vi "prototype_terminal.vi"() -> ()   [LabVIEW 2015]
uses:
  <vilib>/Analysis/baseanly.llb/Mean (DBL).vi
  <vilib>/Instr/_visa.llb/VISA Configure Serial Port (Instr).vi
  <vilib>/Analysis/NI_AALBase.lvlib
panel:
  in  "Tab Control":T1(tab)
  in  "Select channel":T2
  out "Current values":cluster{dbl, dbl, dbl, dbl}(graph)
  out "Error thermometer":bool
  out "Error pressure":bool
  out "Error amperage":bool
  out "Error voltage":bool
  out "SMA":cluster{dbl, dbl, dbl, dbl}(graph)
  in  "Clear":bool
  out "Amperage,A":dbl(slide) scale=0.0..2.5
  out "Pressure, kPa":dbl(knob) scale=0.0..50.0
  out "Thermometer, °C":dbl(slide) scale=0.0..60.0
  out "Voltage,V":dbl(knob) scale=0.0..5.0 scale format="%_2f"
  out "Voltage":dbl(graph)
  in  "Set voltage":sgl(knob) min=1 max=5 step=0.01 scale=0.0..5.0 scale format="%#.2f"
  out "Output voltage,V":dbl(knob) scale=1.0..5.0 scale format="%_2f"
  out "Received bytes":dbl
  in  "VISA resource name":refnum<visa-resource-name>
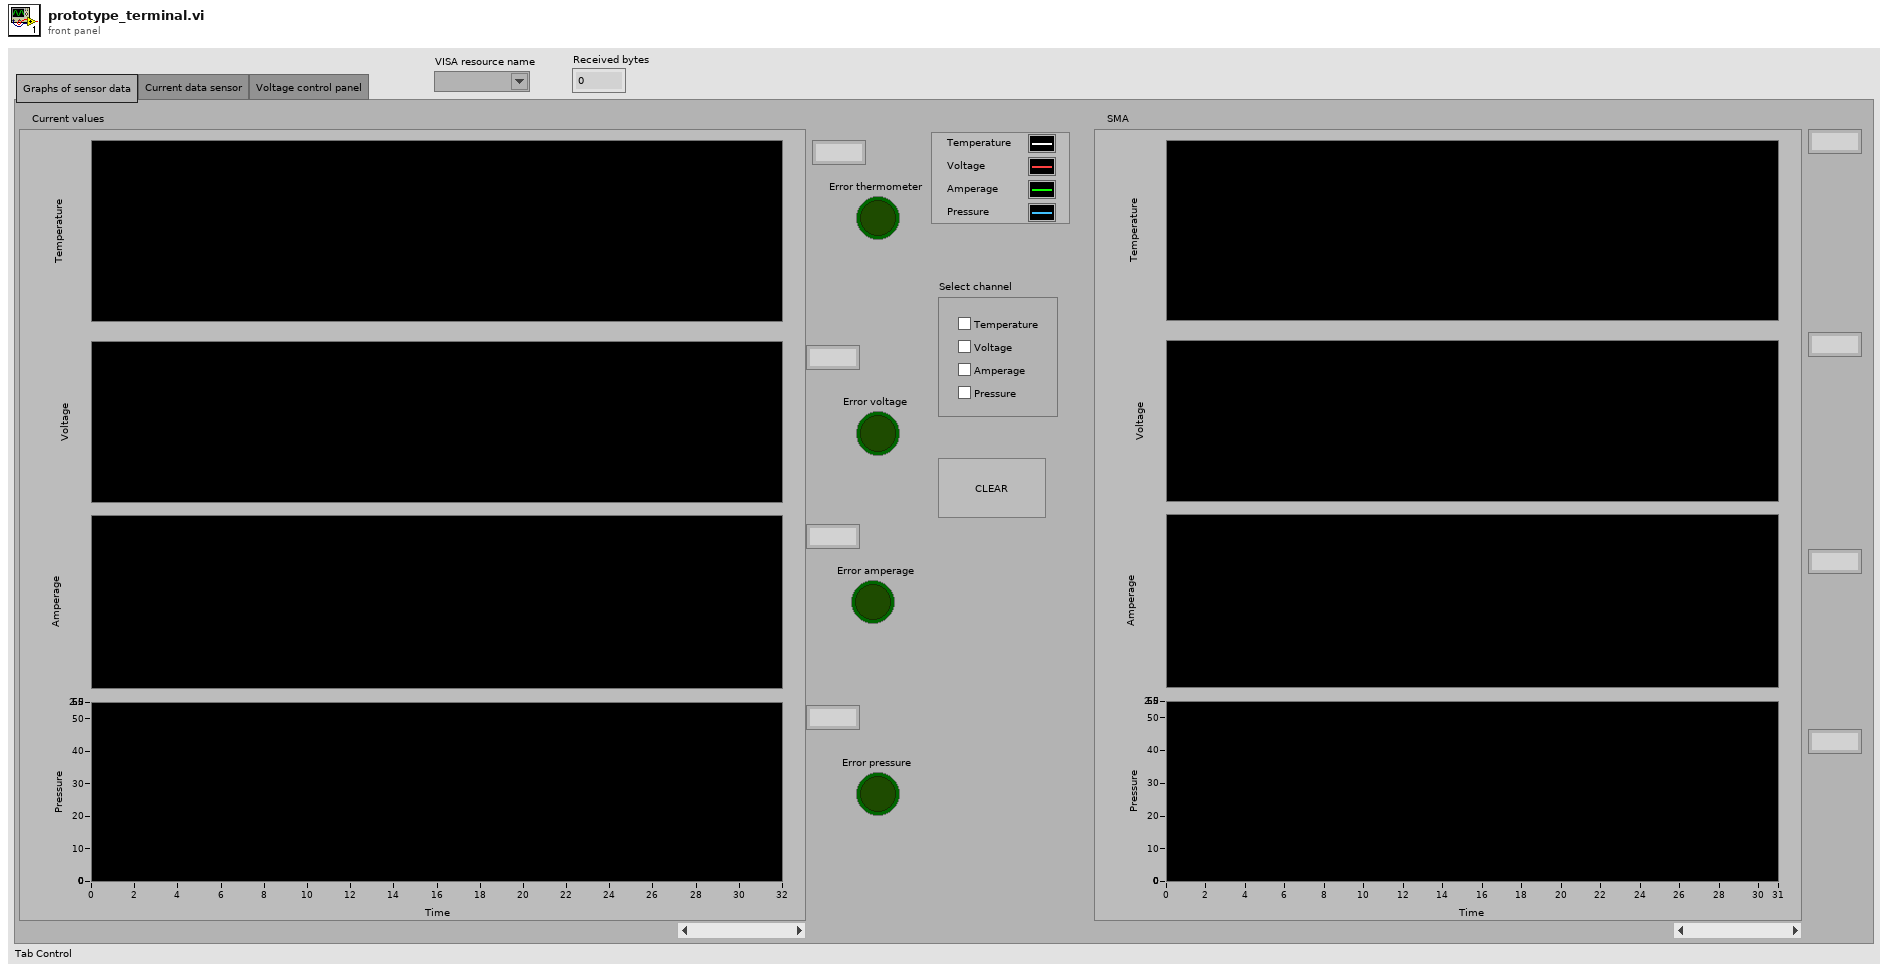
[diagram p1: front panel]
types:
  T1 = enum32{"Graphs of sensor data", "Current data sensor", "Voltage control panel"}
  T2 = cluster{"Ch1":bool, "Ch2":bool, "Ch3":bool, "Ch3 2":bool}
  T3 = cluster{"mean":dbl, "mean":dbl, "mean":dbl, "mean":dbl}
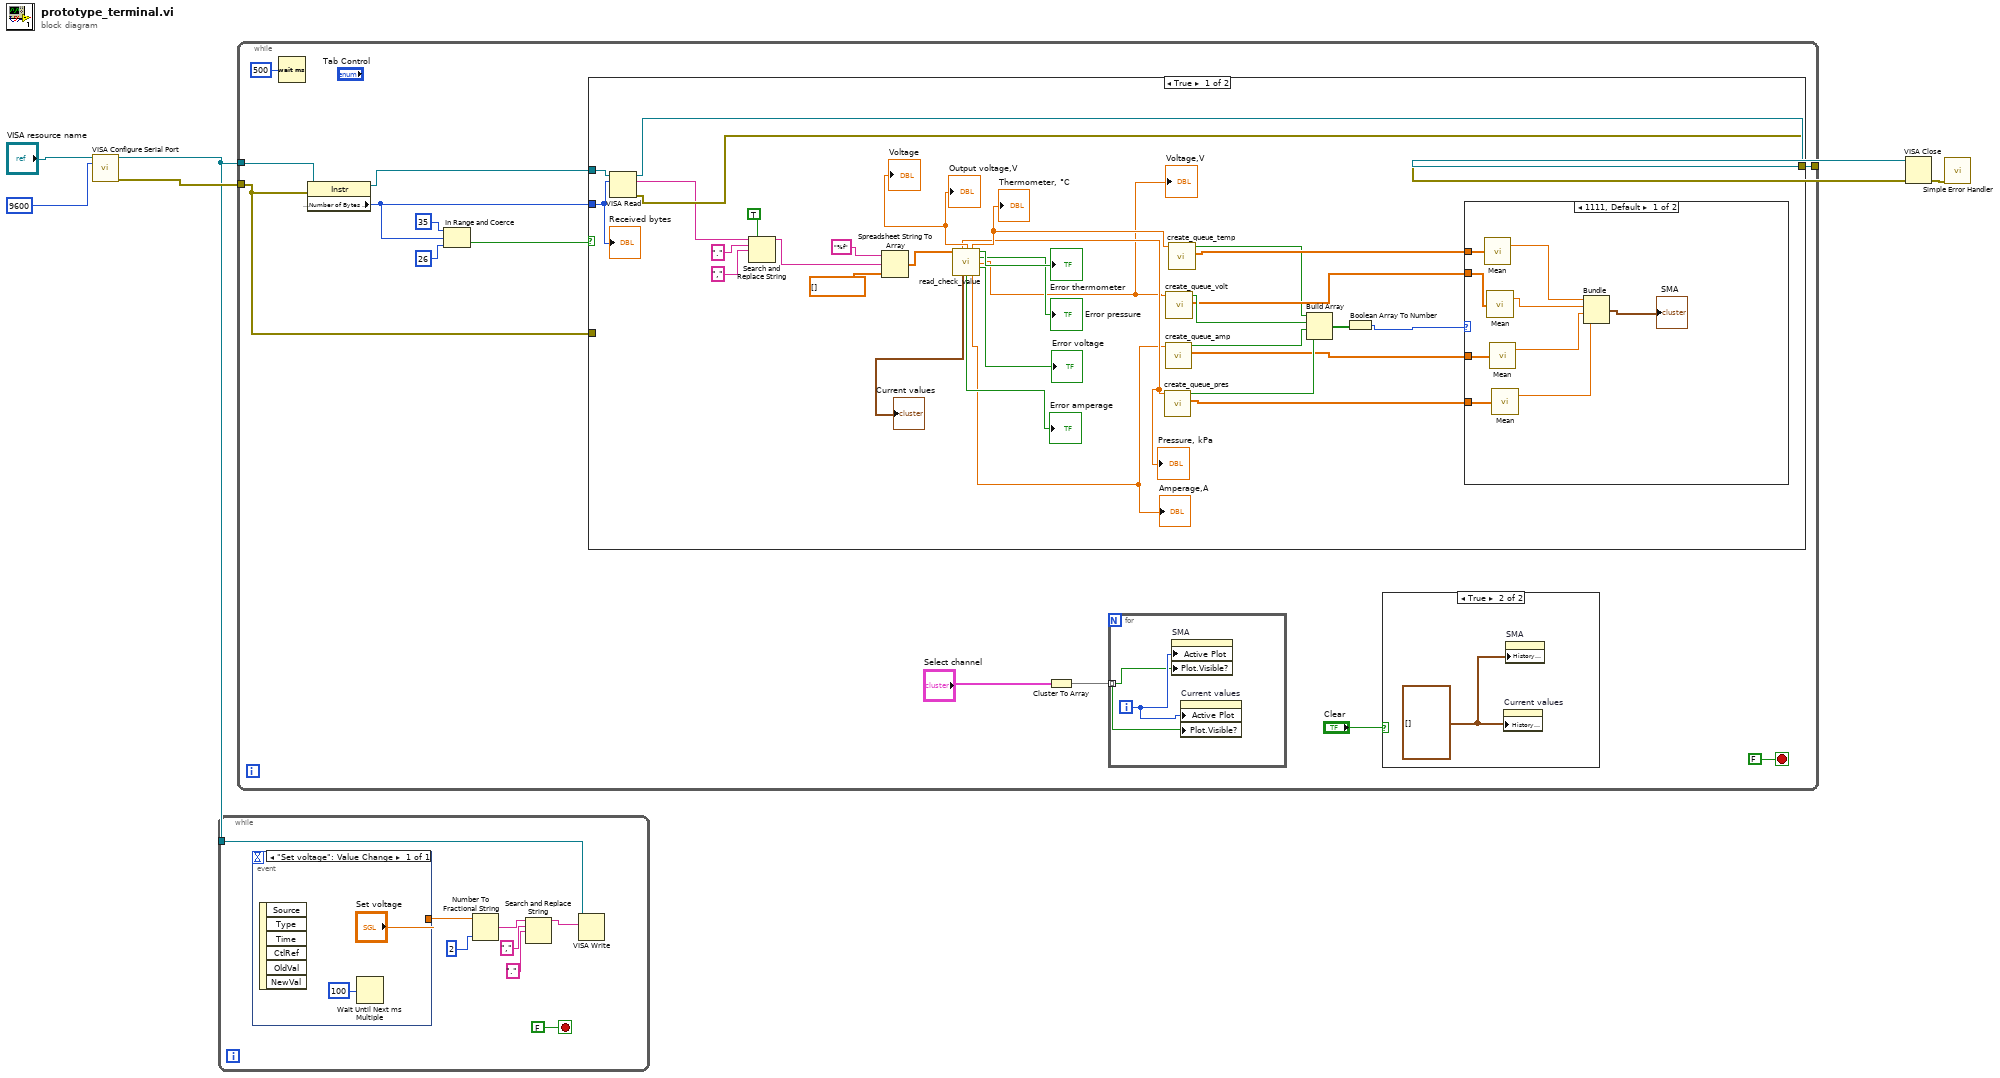
[diagram p0: block diagram]
diagram:
  n1 = call-poly "VISA Configure Serial Port"("VISA resource name"="VISA resource name", "baud rate (9600)"=u32 9600) -> ("VISA resource name out"=w5:refnum<visa-resource-name>, "error out"=w7:errorcluster)  [unwired: 12 in]
  n2 = while {
    tunnel: w5 -> [w12]
    stop <- FALSE stop-if-true
    n3 = event shown="[0] \"Set voltage\": Value Change" {
      selector: _ -> [_]
      dyn-events: _ -> [_]
      timeout: _ -> [_]
      tunnel: ["Set voltage"] -> w13
      event "Set voltage": Value Change {
        n4 = event-data() -> ()  [unwired: 1 in, 6 out]
        n5 = Wait Until Next ms Multiple(millisecond multiple=u32 100) -> ()  [unwired: 1 out]
      }
    }
    n6 = Number To Fractional String(number=w13, precision (6)=i16 2) -> (F-format string=w11:string)  [unwired: 2 in]
    n7 = Search and Replace String(input string=w11, search string=",", replace string="." ("replace string (\"\")")) -> (result string=w10:string)  [unwired: 5 in, 3 out]
    n8 = VISA Write(VISA resource name=w12, write buffer=w10) -> ()  [unwired: 1 in, 3 out]
  }
  n9 = while {
    tunnel: w5 -> [w31]
    tunnel: w7 -> [w28]
    tunnel: [w30] -> w4
    tunnel: [w29] -> w3
    stop <- FALSE stop-if-true
    n10 = Wait (ms)(milliseconds to wait=u32 500) -> ()  [unwired: 1 out]
    n11 = property class="Instr"(reference=w31, error in=w28) -> (reference out=w23:refnum<visa-resource-name>, "Serial Settings:Number of Bytes at Serial Port"=w19:u32)  [unwired: 1 out]
    n12 = In Range and Coerce(upper limit=u32 35, x=w19, lower limit=u32 26) -> (In Range?=w22:bool)  [unwired: 1 out]
    n13 = case shown="True" w22 {
      tunnel: w23 -> [w62 w77]
      tunnel: [w64 w77] -> w30
      tunnel: [w63 w76] -> w29
      tunnel: w28 -> [_ w76]
      tunnel: w19 -> [w61 _]
      frame True {
        n14 = VISA Read(VISA resource name=w62, byte count=w61) -> (VISA resource name out=w64:refnum<visa-resource-name>, read buffer=w52:string, error out=w63:errorcluster)  [unwired: 1 in, 1 out]
        n15 = Search and Replace String(replace all?=TRUE ("replace all? (F)"), input string=w52, search string="." ("replace string (\"\")"), replace string="," ("replace string (\"\")")) -> (result string=w53:string)  [unwired: 4 in, 3 out]
        n16 = Spreadsheet String To Array(format string="%f", spreadsheet string=w53, array type (2D Dbl)=dbl[] []) -> (array=w60:dbl[])  [unwired: 1 in]
        n17 = call "read_check_value.vi"("Array values"=w60) -> ("Pressure"=w37:dbl, "Knob_voltage"=→"Output voltage,V" →"Voltage":dbl, "Temparature"=w38:dbl, "Error thermometer?"=→"Error thermometer":bool, "Error pressure?"=→"Error pressure":bool, "Voltage"=w35:dbl, "Error voltage?"=→"Error voltage":bool, "Cluster of values"=→"Current values":cluster{dbl, dbl, dbl, dbl}, "Error amperage?"=→"Error amperage":bool, "Amperage"=w36:dbl)  [unwired: 5 in]
        "Thermometer, °C" <- w38
        "Amperage,A" <- w36
        "Pressure, kPa" <- w37
        "Voltage,V" <- w35
        n18 = call "create_queue_pres.vi"("Value"=w37) -> ("Current Queue"=w43:dbl[], "Boolean"=w48:bool)  [unwired: 9 in]
        n19 = call "create_queue_amp.vi"("Value"=w36) -> ("Current Queue"=w44:dbl[], "Boolean"=w41:bool)  [unwired: 9 in]
        n20 = call "create_queue_volt.vi"("Value"=w35) -> ("Current Queue"=w45:dbl[], "Boolean"=w49:bool)  [unwired: 9 in]
        n21 = call "create_queue_temp.vi"("Value"=w38) -> ("Current Queue"=w46:dbl[], "Boolean"=w40:bool)  [unwired: 9 in]
        n22 = Build Array(w40, w49, w41, w48) -> (w47:bool[])
        n23 = Boolean Array To Number(Boolean array=w47) -> (number=w42:u32)
        n24 = case shown="1111, Default" w42 {
          tunnel: w46 -> [w75 _]
          tunnel: w45 -> [w74 _]
          tunnel: w44 -> [w73 _]
          tunnel: w43 -> [w72 _]
          frame 15, Default {
            n25 = call-poly <vilib>:"Mean.vi"("X"=w75) -> ("mean"=w71:dbl)  [unwired: 1 out]
            n26 = call-poly <vilib>:"Mean.vi"("X"=w74) -> ("mean"=w70:dbl)  [unwired: 1 out]
            n27 = call-poly <vilib>:"Mean.vi"("X"=w73) -> ("mean"=w69:dbl)  [unwired: 1 out]
            n28 = call-poly <vilib>:"Mean.vi"("X"=w72) -> ("mean"=w68:dbl)  [unwired: 1 out]
            n29 = Bundle("mean"=w71, "mean"=w70, "mean"=w69, "mean"=w68) -> (→"SMA":T3)  [unwired: 1 out]
          }
          frame 0 {
          }
        }
        "Received bytes" <- w61
      }
      frame False {
      }
    }
    n30 = Cluster To Array(cluster="Select channel") -> (array=w25:bool[])
    n31 = for {
      tunnel: w25 -> [w32] mode=indexing
      i -> [w33]
      n32 = property on="SMA" class="WFChart (strict)"("Active Plot"=w33, "Plot.Visible?"=w32) -> ()  [unwired: 2 in, 2 out]
      n33 = property on="Current values" class="WFChart (strict)"("Active Plot"=w33, "Plot.Visible?"=w32) -> ()  [unwired: 2 in, 2 out]
    }
    n34 = case shown="True" "Clear" {
      frame False {
      }
      frame True {
        w34 = cluster{dbl, dbl, dbl, dbl}[] [] ("History Data")
        n35 = property on="Current values" class="WFChart (strict)"("History Data"=w34) -> ()  [unwired: 2 in, 2 out]
        n36 = property on="SMA" class="WFChart (strict)"("History Data"=w34) -> ()  [unwired: 2 in, 2 out]
      }
    }
  }
  n37 = VISA Close(VISA resource name=w4, error in (no error)=w3) -> (error out=w6:errorcluster)
  n38 = call <vilib>:"Simple Error Handler.vi"("error in (no error)"=w6) -> ()  [unwired: 4 in, 5 out]
